vi "PVcam_consumer.vi"(11 "?":T3) -> ()   [LabVIEW 2025]
uses:
  support/Message Queue/Messsage cues to camera.ctl
  support/Message Queue/Message Cluster_TICO behavior.ctl
  camera parameters.ctl
  <vilib>/vision/Image Controls.llb/IMAQ Image.ctl
  camera parameter message cluster.ctl
  support/Message Queue/Enqueue Message (Single)_TICO behavior.vi
panel:
  in  "Image scale":cluster{dbl, dbl}(slide)={0.0, 2.4242424242424243} scale=0.0..10.0
  out "display auto exposure":dbl
  in  "Change camera mode 2":bool
  in  "exposure time (µs)":dbl=1.0 min=1.0 max=2400.0 step=1.0
  in  "H":dbl=1.0 min=1.0 max=2400.0 step=1.0
  in  "W":dbl=1.0 min=1.0 max=2400.0 step=1.0
  in  "Y":dbl=1.0 min=1.0 max=2400.0 step=1.0
  in  "X":dbl=1.0 min=1.0 max=2400.0 step=1.0
  out "H 2":dbl=1.0 caption="H" min=1.0 max=2400.0 step=1.0
  out "W 2":dbl=1.0 caption="W" min=1.0 max=2400.0 step=1.0
  out "X 2":dbl=1.0 caption="Y" min=1.0 max=2400.0 step=1.0
  out "Y 2":dbl=1.0 caption="X" min=1.0 max=2400.0 step=1.0
  out "is running":bool
  out "camera mode":string
  in  "Change camera mode":bool
  in  "Cluster":T1
  in  "center FOV":bool
  in  "Default FOV":bool
  in  "Apply ROI":bool
  out "Image":T2(plugin-control)
  # "ROI"
  # "current FOV"
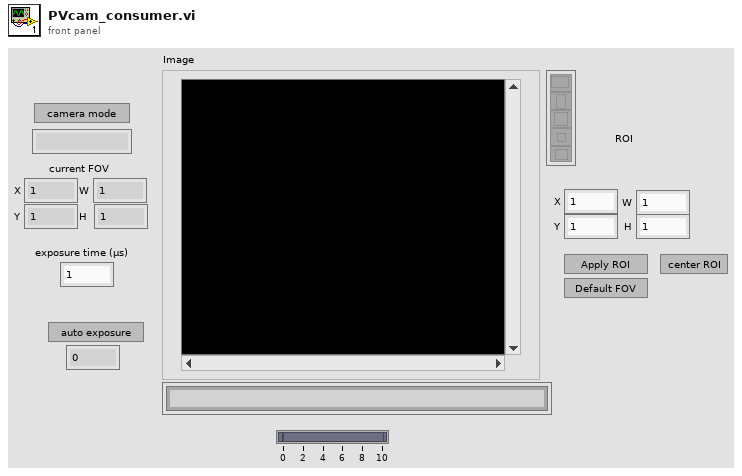
[diagram p1: front panel]
types:
  T1 = typedef "camera parameters.ctl" = cluster{"exposure time (ms)":i32, "FOV":i32[]}
  T2 = typedef "IMAQ Image.ctl" = refnum<image>
  T3 = typedef "Messsage cues to camera.ctl" = cluster{"Camera Queue":refnum<queue>, "Stop Queue ":refnum<queue>}
  T4 = typedef "Camera Description.ctl" = cluster{"Serial Number":string, "Chip Name":string, "Sensor Width":u32, "Sensor Height":u32, "Firmware version":string, "Interface":string, "Part Number":string, "Product Name":string}
  T5 = cluster{"Camera 0 Name ":string, "Camera Description":T4}
  T6 = typedef "camera parameter message cluster.ctl" = cluster{"parameter":string, "single value":i32, "Array value":dbl[]}
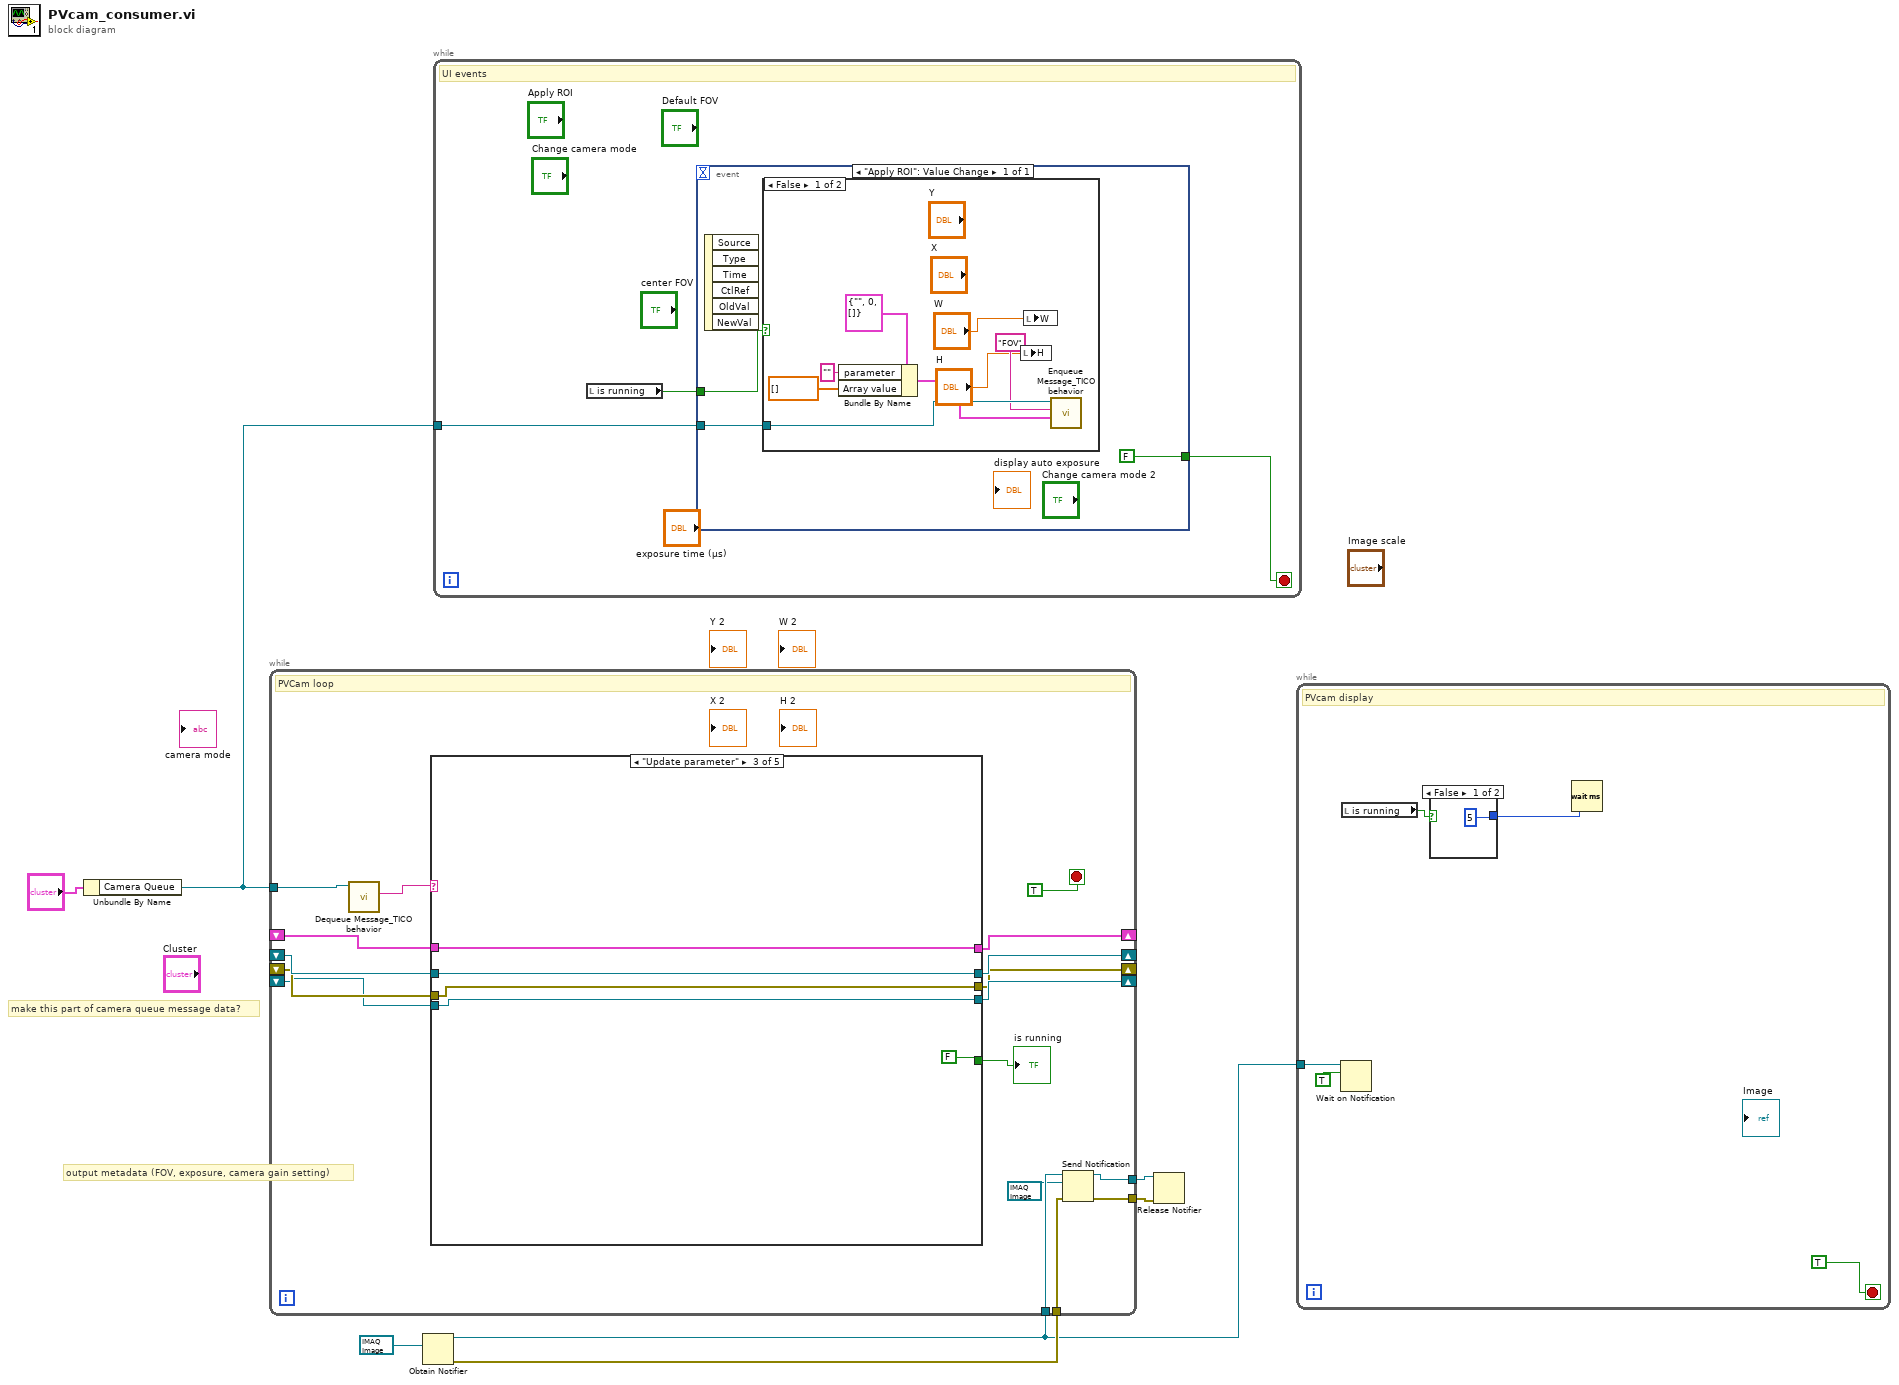
[diagram p0: block diagram]
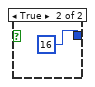
[diagram p3: hidden frame]
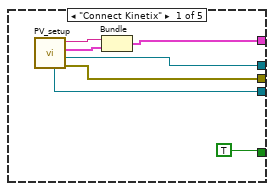
[diagram p4: hidden frame]
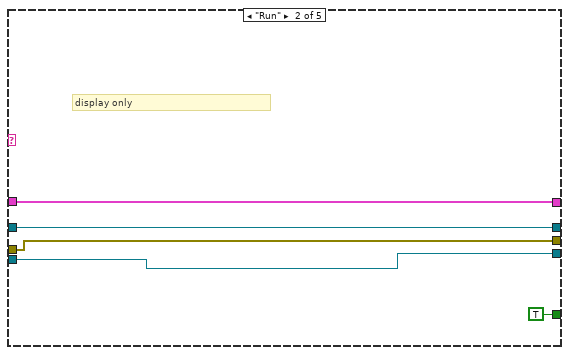
[diagram p5: hidden frame]
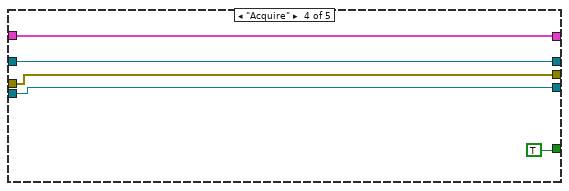
[diagram p6: hidden frame]
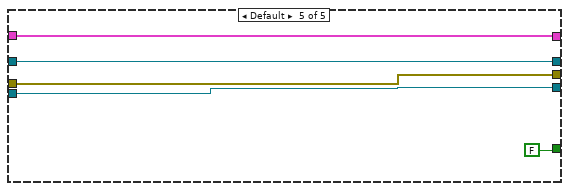
[diagram p7: hidden frame]
diagram:
  # "output metadata (FOV, exposure, camera gain setting)"
  # "make this part of camera queue message data?"
  n1 = Unbundle By Name("?") -> ("Camera Queue"=w2:refnum<queue>)
  n2 = Obtain Notifier(notification data type=T2 refnum ("Image")) -> (notifier out=w1:refnum<notifier>, error out=w4:errorcluster)  [unwired: 3 in, 1 out]
  n3 = while {
    shift-right: [w23] -> _
    shift-left: _ -> [w19]
    shift-right: [w21] -> _
    shift-left: _ -> [w18]
    shift-right: [w20] -> _
    shift-left: _ -> [w17]
    shift-right: [w22] -> _
    shift-left: _ -> [w16]
    tunnel: [w14] -> w6
    tunnel: [w13] -> w5
    tunnel: w4 -> [w12]
    tunnel: w2 -> [w11]
    tunnel: w1 -> [w9]
    stop <- TRUE stop-if-true
    # "PVCam loop"
    n4 = call "Dequeue Message_TICO behavior.vi"("Message Queue"=w11) -> ("Message"=w15:string)  [unwired: 7 in, 3 out]
    n5 = case shown="\"Update parameter\"" w15 {
      tunnel: [w29 w36 w40 w46 w51] -> w23
      tunnel: [w28 w33 w39 w45 w50] -> w21
      tunnel: [w27 w34 w38 w44 w49] -> w20
      tunnel: [w26 w35 w37 w43 w48] -> w22
      tunnel: w19 -> [_ w36 w40 w46 w51]
      tunnel: w18 -> [_ w33 w39 w45 w50]
      tunnel: w17 -> [_ w34 w38 w44 w49]
      tunnel: w16 -> [_ w35 w37 w43 w48]
      tunnel: [TRUE ("is running") TRUE ("is running") FALSE ("is running") TRUE ("is running") FALSE ("is running")] -> w10
      frame "Connect Kinetix" {
        n6 = call "PV_setup.vi"() -> ("error out"=w27:errorcluster, "Camera out"=w28:refnum<class "Camera.lvclass">, "Camera Description"=w30:T4, "Camera 0 Name"=w31:string, "PVCAM Out"=w26:refnum<class "PVCAM.lvclass">)  [unwired: 7 in]
        n7 = Bundle("Camera 0 Name"=w31, "Camera Description"=w30) -> (w29:T5)  [unwired: 1 in]
      }
      frame "Run" {
        # "display only"
      }
      frame "Update parameter" {
      }
      frame "Acquire" {
      }
      frame Default {
      }
    }
    "is running" <- w10
    n8 = Send Notification(notification=T2 refnum, notifier=w9, error in (no error)=w12) -> (notifier out=w14:refnum<notifier>, error out=w13:errorcluster)
  }
  n9 = while {
    tunnel: w2 -> [w54]
    stop <- w52 stop-if-true
    # "UI events"
    n10 = local read "is running"() -> (w53:bool)
    n11 = event shown="[0] \"Apply ROI\": Value Change" {
      selector: _ -> [_]
      dyn-events: _ -> [_]
      timeout: _ -> [_]
      tunnel: w54 -> [w57]
      tunnel: w53 -> [w56]
      tunnel: [FALSE] -> w52
      event "Apply ROI": Value Change {
        n12 = event-data() -> ()  [unwired: 1 in, 6 out]
        n13 = case shown="False" w56 {
          tunnel: w57 -> [w65 _]
          frame False {
            n14 = Bundle By Name(cluster=T6 {"parameter"="", "single value"=0, "Array value"=[]}, "parameter"="", "Array value"=dbl[] []) -> (w63:T6)
            n15 = local write "H"("H") -> ()
            n16 = local write "W"("W") -> ()
            n17 = call-poly "Enqueue Message_TICO behavior.vi"("Message Data"=w63, "Message"="FOV", "Message Queue"=w65) -> ()  [unwired: 7 in, 2 out]
          }
          frame True {
          }
        }
      }
    }
  }
  n18 = Release Notifier(notifier=w6, error in (no error)=w5) -> ()  [unwired: 1 in, 3 out]
  n19 = while {
    tunnel: w1 -> [w69]
    stop <- TRUE stop-if-true
    # "PVcam display"
    n20 = Wait on Notification(notifier=w69, ignore previous (F)=TRUE) -> ()  [unwired: 2 in, 4 out]
    n21 = local read "is running"() -> (w67:bool)
    n22 = case shown="False" w67 {
      tunnel: [u32 5 ("milliseconds to wait") u32 16 ("milliseconds to wait")] -> w66
      frame False {
      }
      frame True {
      }
    }
    n23 = Wait (ms)(milliseconds to wait=w66) -> ()  [unwired: 1 out]
  }
